vi "HEWH InitializeEquipmet.vi"(7 "Semiphore":T1, 8 "Error In":errorcluster, 9 "GEA2?":bool, 10 "Agilent Channel Input":string, 11 "Equipment":T3={"COM Port"="COM1", "MW100"="MW100", "AG34970"="A-34972A", "Chamber"="WT500"}) -> (0 "Error Out":errorcluster, 1 "Computer Name":string, 2 "LAN IP Address":string, 3 "Equipment Out":T3={"COM Port"="COM1", "MW100"="MW100", "AG34970"="A-34972A", "Chamber"="WT500"})   [LabVIEW 2012]
uses:
  EquipReferences.ctl
  <vilib>/Instr/_visa.llb/VISA Configure Serial Port (Instr).vi
  Drivers/Agilent 34970/Agilent 34970.lvlib
  <vilib>/Utility/config.llb/NI_LVConfig.lvlib
panel:
  in  "Retries":i32=1
  in  "Target IP Address":string
  out "error cluster":T2
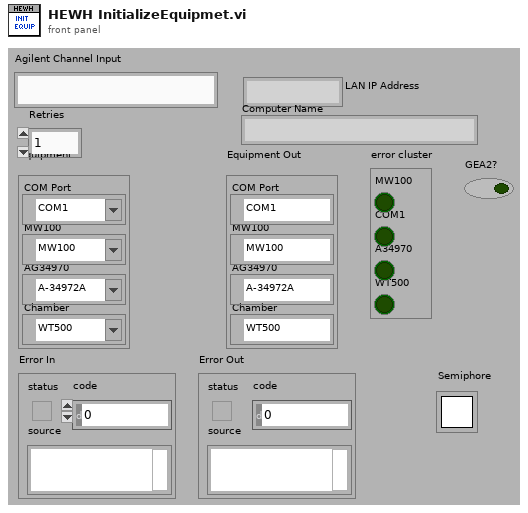
[diagram p1: front panel]
types:
  T1 = typedef "Semaphore RefNum" = refnum<k1>
  T2 = cluster{"MW100":bool, "COM1":bool, "A34970":bool, "WT500":bool}
  T3 = typedef "EquipReferences.ctl" = cluster{"COM Port":refnum<visa-resource-name>, "MW100":refnum<visa-resource-name>, "AG34970":refnum<visa-resource-name>, "Chamber":refnum<visa-resource-name>}
  T4 = enum16{"Computation Start", "Computation stop", "Reset Computation", "Clear Computation"}
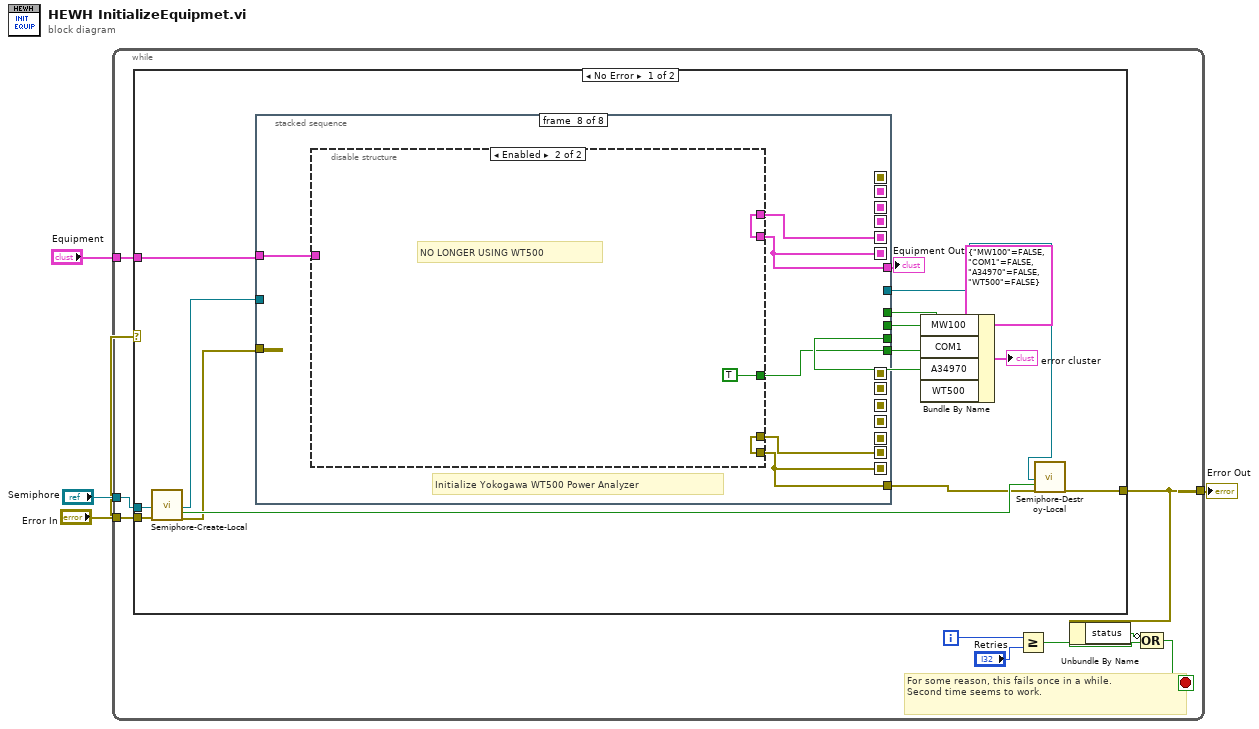
[diagram p0: block diagram]
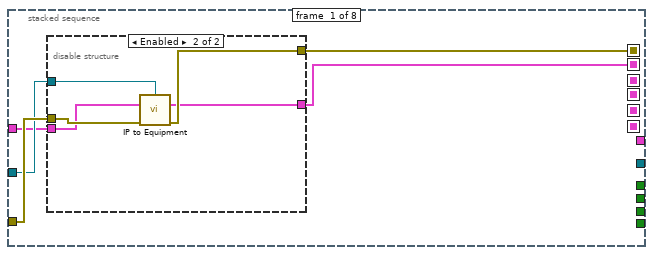
[diagram p2: hidden frame]
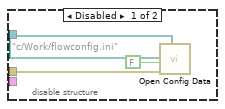
[diagram p3: hidden frame]
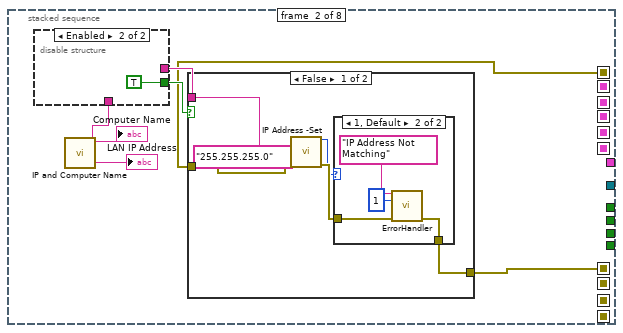
[diagram p4: hidden frame]
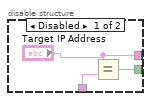
[diagram p5: hidden frame]
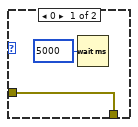
[diagram p6: hidden frame]
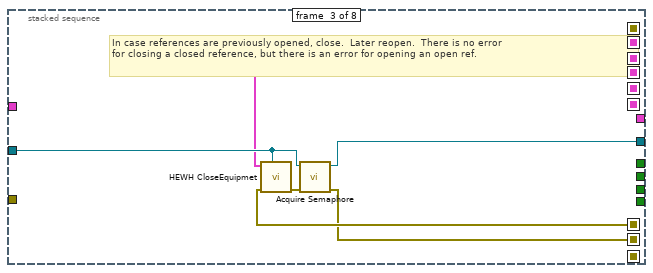
[diagram p8: hidden frame]
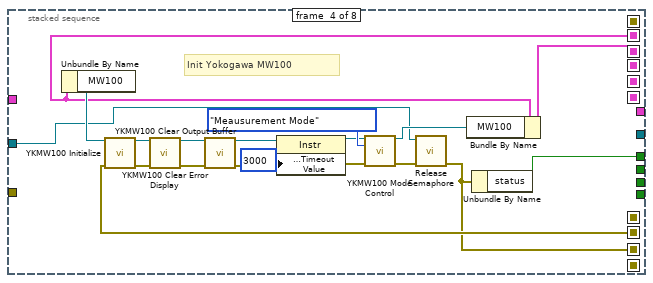
[diagram p9: hidden frame]
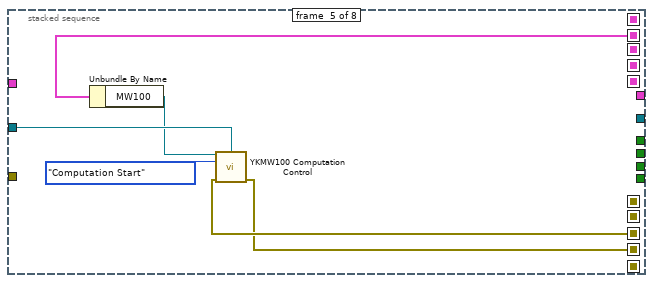
[diagram p10: hidden frame]
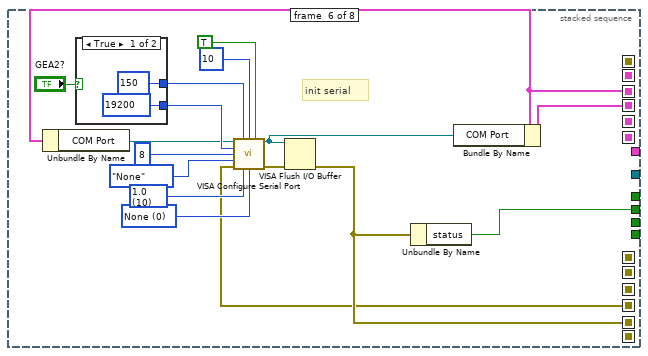
[diagram p11: hidden frame]
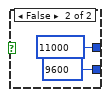
[diagram p12: hidden frame]
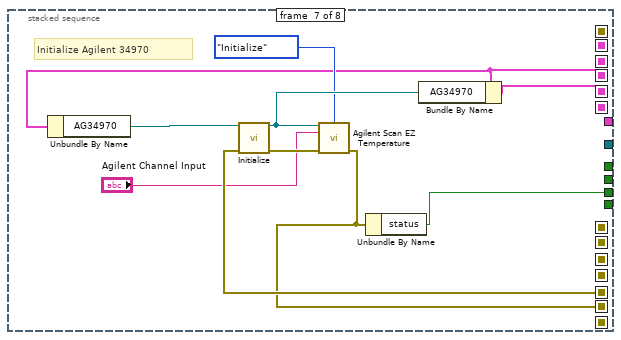
[diagram p13: hidden frame]
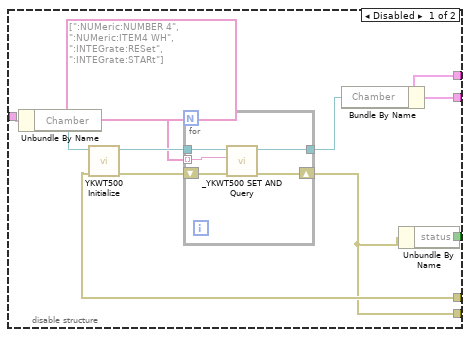
[diagram p14: hidden frame]
diagram:
  n1 = while {
    tunnel: "Equipment" -> [w13]
    tunnel: "Semiphore" -> [w12]
    tunnel: [w7] -> w2
    tunnel: "Error In" -> [w11]
    i -> [w10]
    stop <- w5 stop-if-true
    # "For some reason, this fails once in a while.\nSecond time seems to work."
    n2 = case shown="No Error" w11 {
      tunnel: w13 -> [w22 _]
      tunnel: w12 -> [w21 _]
      tunnel: w11 -> [w19 w153]
      tunnel: [w18 w153] -> w7
      frame No Error {
        n3 = call "Semiphore-Create-Local.vi"("Semiphore"=w21, "error in (no error)"=w19) -> ("semaphore"=w16:T1, "Local?"=w20:bool, "error out"=w17:errorcluster)  [unwired: 15 in]
        n4 = stacked-sequence {
          seq-local: [_ _ _ w73 _ _ _ _] -> [_ _ _ _ w96 _ _ _]
          seq-local: [_ _ _ _ _ w101 _ _] -> [_ _ _ _ _ _ w125 _]
          seq-local: [_ _ _ w89 _ _ _ _] -> [_ _ _ _ w91 w97 _ _]
          seq-local: [_ _ _ _ _ w106 _ _] -> [_ _ _ _ _ _ w118 _]
          seq-local: [_ _ _ _ _ _ w127 _] -> [_ _ _ _ _ _ _ w132]
          seq-local: [_ _ _ _ _ _ w123 _] -> [_ _ _ _ _ _ _ w131]
          seq-local: [_ _ _ _ _ _ _ w130] -> [_ _ _ _ _ _ _ _]
          seq-local: [_ _ _ _ _ _ _ w128] -> [_ _ _ _ _ _ _ _]
          seq-local: [_ w47 _ _ _ _ _ _] -> [_ _ w69 _ _ _ _ _]
          seq-local: [_ _ w68 _ _ _ _ _] -> [_ _ _ w77 _ _ _ _]
          seq-local: [_ _ _ _ w95 _ _ _] -> [_ _ _ _ _ w99 _ _]
          seq-local: [w33 _ _ _ _ _ _ _] -> [_ w43 _ _ _ _ _ _]
          seq-local: [w30 _ _ _ _ _ _ _] -> [_ _ w66 w72 _ _ _ _]
          tunnel: w17 -> [w34 _ _ _ _ _ _ _]
          tunnel: w22 -> [w31 _ _ _ _ _ _ w133]
          tunnel: [_ _ _ _ _ _ _ w130] -> w29
          tunnel: [_ _ _ _ _ _ _ w128] -> w14
          tunnel: [_ _ _ w88 _ _ _ _] -> w28
          tunnel: [_ _ _ _ _ w104 _ _] -> w27
          tunnel: [_ _ _ _ _ _ w124 _] -> w26
          tunnel: [_ _ _ _ _ _ _ w129] -> w25
          tunnel: w16 -> [w32 _ w70 w74 w94 _ _ _]
          tunnel: [_ _ w67 _ _ _ _ _] -> w15
          frame #0 {
            n5 = disable-structure shown="Enabled" {
              disable-tunnel: w34 -> [w36 w42]
              disable-tunnel: [_ w41] -> w33
              disable-tunnel: w32 -> [_ w40]
              disable-tunnel: w31 -> [_ w39]
              disable-tunnel: [_ w38] -> w30
              frame Disabled {
                n6 = call <vilib>:"Open Config Data.vi"("error in (no error)"=w36, "create file if necessary (T)"=FALSE, "configuration file path"=path "c:/Work/flowconfig.ini") -> ()  [unwired: 6 in, 3 out]
              }
              frame Enabled {
                n7 = call "IP to Equipment.vi"("MW100 Semiphore"=w40, "Equipment In"=w39, "Error In"=w42) -> ("Equipment Out"=w38:T3, "Error Out"=w41:errorcluster)  [unwired: 10 in, 1 out]
              }
            }
          }
          frame #1 {
            n8 = call "IP and Computer Name.vi"() -> ("IP Address"=w48:string, "Computer Name"=→"Computer Name":string)  [unwired: 10 in]
            "LAN IP Address" <- w48
            n9 = disable-structure shown="Enabled" {
              disable-tunnel: w48 -> [w51 _]
              disable-tunnel: [w50 TRUE] -> w46
              disable-tunnel: ["Target IP Address" _] -> w45
              frame Disabled {
                n10 = Equal?(x="Target IP Address", y=w51) -> (x = y?=w50:bool)
              }
              frame Enabled {
              }
            }
            n11 = case shown="False" w46 {
              tunnel: [w58 w65] -> w47
              tunnel: w43 -> [w55 w65]
              tunnel: w45 -> [w56 _]
              frame False {
                n12 = call "IP Address -Set.vi"("IP Address"=w56, "Submet Mask"="255.255.255.0", "error in (no error)"=w55) -> ("return code"=w53:i32, "error out"=w54:errorcluster)  [unwired: 9 in, 2 out]
                n13 = case shown="1, Default" w53 {
                  tunnel: [w60 w64] -> w58
                  tunnel: w54 -> [w60 w61]
                  frame 0 {
                    n14 = Wait (ms)(milliseconds to wait=u32 5000) -> ()  [unwired: 1 out]
                  }
                  frame 1, Default {
                    n15 = call "ErrorHandler.vi"("Error Message"="IP Address Not Matching", "code"=1, "Error In"=w61) -> ("Error Out"=w64:errorcluster)  [unwired: 12 in]
                  }
                }
              }
              frame True {
              }
            }
          }
          frame #2 {
            # "In case references are previously opened, close.  Later reopen.  There is no error\nfor closing a closed reference, but there is an error for opening an open ref."
            n16 = call "HEWH CloseEquipmet.vi"("Semiphore"=w70, "Error In"=w69, "Equipment"=w66) -> ("Error Out"=w71:errorcluster)  [unwired: 8 in]
            n17 = call <vilib>:"Acquire Semaphore.vi"("error in (no error)"=w71, "semaphore"=w70) -> ("error out"=w68:errorcluster, "semaphore out"=w67:T1)  [unwired: 3 in, 1 out]
          }
          frame #3 {
            # "Init Yokogawa MW100"
            n18 = Unbundle By Name(w72) -> ("MW100"=w90:refnum<visa-resource-name>)
            n19 = call "YKMW100 Initialize.vi"("VISA session (TCPIP::)"=w90, "error in (no error)"=w77) -> ("dup VISA session"=w78:refnum<visa-resource-name>, "error out"=w81:errorcluster)  [unwired: 12 in]
            n20 = call "YKMW100 Clear Error Display.vi"("VISA session"=w78, "error in (no error)"=w81) -> ("dup VISA session"=w79:refnum<visa-resource-name>, "error out"=w80:errorcluster)  [unwired: 10 in, 2 out]
            n21 = call "YKMW100 Clear Output Buffer.vi"("VISA session"=w79, "error in (no error)"=w80) -> ("dup VISA session"=w82:refnum<visa-resource-name>, "error out"=w83:errorcluster)  [unwired: 12 in]
            n22 = property class="Instr"(reference=w82, error in=w83, "General Settings:Timeout Value"=u32 3000) -> (reference out=w84:refnum<visa-resource-name>, error out=w85:errorcluster)
            n23 = call "YKMW100 Mode Control.vi"("VISA session"=w84, "Model"=enum16{"Meausurement Mode", "Setting Mode"}."Meausurement Mode", "error in (no error)"=w85) -> ("dup VISA session"=w76:refnum<visa-resource-name>, "error out"=w75:errorcluster)  [unwired: 11 in]
            n24 = call <vilib>:"Release Semaphore.vi"("error in (no error)"=w75, "semaphore"=w74) -> ("error out"=w73:errorcluster)  [unwired: 4 in, 1 out]
            n25 = Bundle By Name(cluster=w72, "MW100"=w76) -> (w89:T3)
            n26 = Unbundle By Name(w73) -> ("status"=w88:bool)
          }
          frame #4 {
            n27 = Unbundle By Name(w91) -> ("MW100"=w93:refnum<visa-resource-name>)
            n28 = call "YKMW100 Computation Control.vi"("VISA session"=w93, "Semiphore"=w94, "Mode"=T4."Computation Start", "error in (no error)"=w96) -> ("error out"=w95:errorcluster)  [unwired: 10 in, 1 out]
          }
          frame #5 {
            w109 = u16 0 items=["None", "XON/XOFF", "RTS/CTS", "XON/XOFF & RTS/CTS", "DTR/DSR", "XON/XOFF & DTR/DSR"] ("flow control (0:none)")
            w110 = u16 10 items=["1.0"=10, "1.5"=15, "2.0"=20] ("stop bits (10: 1 bit)")
            # "init serial"
            n29 = Unbundle By Name(w97) -> ("COM Port"=w105:refnum<visa-resource-name>)
            n30 = case shown="True" "GEA2?" {
              tunnel: [u32 19200 ("baud rate (9600)") u32 9600 ("baud rate (9600)")] -> w113
              tunnel: [u32 150 ("timeout (10sec)") u32 11000 ("timeout (10sec)")] -> w103
              frame True {
              }
              frame False {
              }
            }
            n31 = call-poly "VISA Configure Serial Port"("VISA resource name"=w105, "timeout (10sec)"=w103, "termination char\n(0xA = '\\n' = LF)"=u8 10 ("termination char\n(0xA = '\\n' = LF)"), "Enable Termination\nChar (T)"=TRUE ("Enable Termination\nChar (T)"), "baud rate (9600)"=w113, "data bits (8)"=u16 8, "parity (0:none)"=enum16{"None", "Odd", "Even", "Mark", "Space"}."None", "error in (no error)"=w99, "stop bits (10: 1 bit)"=w110, "flow control (0:none)"=w109) -> ("VISA resource name out"=w100:refnum<visa-resource-name>, "error out"=w102:errorcluster)  [unwired: 4 in]
            n32 = VISA Flush I/O Buffer(VISA resource name=w100, error in (no error)=w102) -> (error out=w101:errorcluster)  [unwired: 1 in, 1 out]
            n33 = Unbundle By Name(w101) -> ("status"=w104:bool)
            n34 = Bundle By Name(cluster=w97, "COM Port"=w100) -> (w106:T3)
          }
          frame #6 {
            # "Initialize Agilent 34970"
            n35 = Unbundle By Name(w118) -> ("AG34970"=w126:refnum<visa-resource-name>)
            n36 = call "Initialize.vi"("VISA Resource Name"=w126, "error in (no error)"=w125) -> ("VISA Resource Name Out"=w121:refnum<visa-resource-name>, "error out"=w122:errorcluster)  [unwired: 12 in]
            n37 = call "Agilent Scan EZ Temperature.vi"("VISA Resource Name"=w121, "Control"=enum16{"Initialize", "Read", "Experiment"}."Initialize", "Channel Input"="Agilent Channel Input", "error in (no error)"=w122) -> ("error out"=w123:errorcluster)  [unwired: 8 in, 3 out]
            n38 = Unbundle By Name(w123) -> ("status"=w124:bool)
            n39 = Bundle By Name(cluster=w118, "AG34970"=w121) -> (w127:T3)
          }
          frame #7 {
            # "Initialize Yokogawa WT500 Power Analyzer"
            n40 = disable-structure shown="Enabled" {
              disable-tunnel: w133 -> [w144 _]
              disable-tunnel: w132 -> [w142 w152]
              disable-tunnel: w131 -> [w141 w151]
              disable-tunnel: [w140 w152] -> w130
              disable-tunnel: [w139 TRUE ("status")] -> w129
              disable-tunnel: [w137 w151] -> w128
              frame Disabled {
                n41 = Unbundle By Name(w144) -> ("Chamber"=w143:refnum<visa-resource-name>)
                n42 = call "YKWT500 Initialize.vi"("error in (no error)"=w141, "VISA resource name"=w143) -> ("error out"=w138:errorcluster, "VISA resource name out"=w136:refnum<visa-resource-name>)  [unwired: 7 in, 1 out]
                n43 = for {
                  shift-right: [w148] -> w137
                  shift-left: w138 -> [w149]
                  tunnel: w136 -> [w147]
                  tunnel: [w146] -> w135
                  tunnel: string[] [":NUMeric:NUMBER 4", ":NUMeric:ITEM4 WH", ":INTEGrate:RESet", ":INTEGrate:STARt"] -> [w145] mode=indexing
                  n44 = call "_YKWT500 SET AND Query.vi"("error in (no error)"=w149, "Write Data"=w145, "VISA resource name"=w147) -> ("error out"=w148:errorcluster, "VISA resource name out"=w146:refnum<visa-resource-name>)  [unwired: 5 in, 2 out]
                }
                n45 = Bundle By Name(cluster=w142, "Chamber"=w135) -> (w140:T3)
                n46 = Unbundle By Name(w137) -> ("status"=w139:bool)
              }
              frame Enabled {
                # "NO LONGER USING WT500"
              }
            }
          }
        }
        "Equipment Out" <- w29
        n47 = Bundle By Name(cluster=T2 {"MW100"=FALSE, "COM1"=FALSE, "A34970"=FALSE, "WT500"=FALSE} ("input cluster"), "MW100"=w28, "COM1"=w27, "A34970"=w26, "WT500"=w25) -> (→"error cluster":T2)
        n48 = call "Semiphore-Destroy-Local.vi"("Semiphore"=w15, "Local?"=w20, "error in (no error)"=w14) -> ("error out"=w18:errorcluster)  [unwired: 16 in]
      }
      frame Error {
      }
    }
    n49 = Greater Or Equal?(x=w10, y="Retries") -> (x >= y?=w6:bool)
    n50 = Unbundle By Name(w7) -> ("status"=w8:bool)
    n51 = Compound Arithmetic op=OR(invert w8, w6) -> (w5:bool)
  }
  "Error Out" <- w2
